vi "Connect Initialize APIs.vi"(0 "Logic VI Ref":refnum<vi>, 5 "SubVIs":refnum<vi>[](array[refnum]), 11 "error in (no error)":errorcluster) -> (15 "error out":errorcluster)   [LabVIEW 2021, in "Migrator.lvlib"]
uses:
  Migrator.lvlib
  Migrator Reusables/Migrator Reusables.lvlib
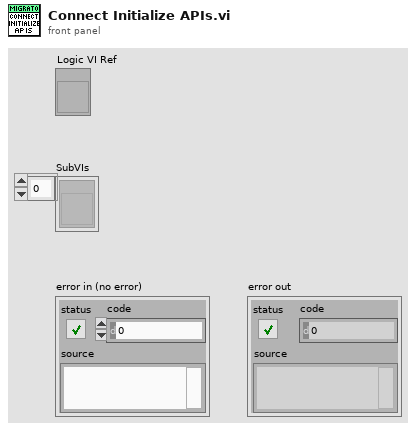
[diagram p1: front panel]
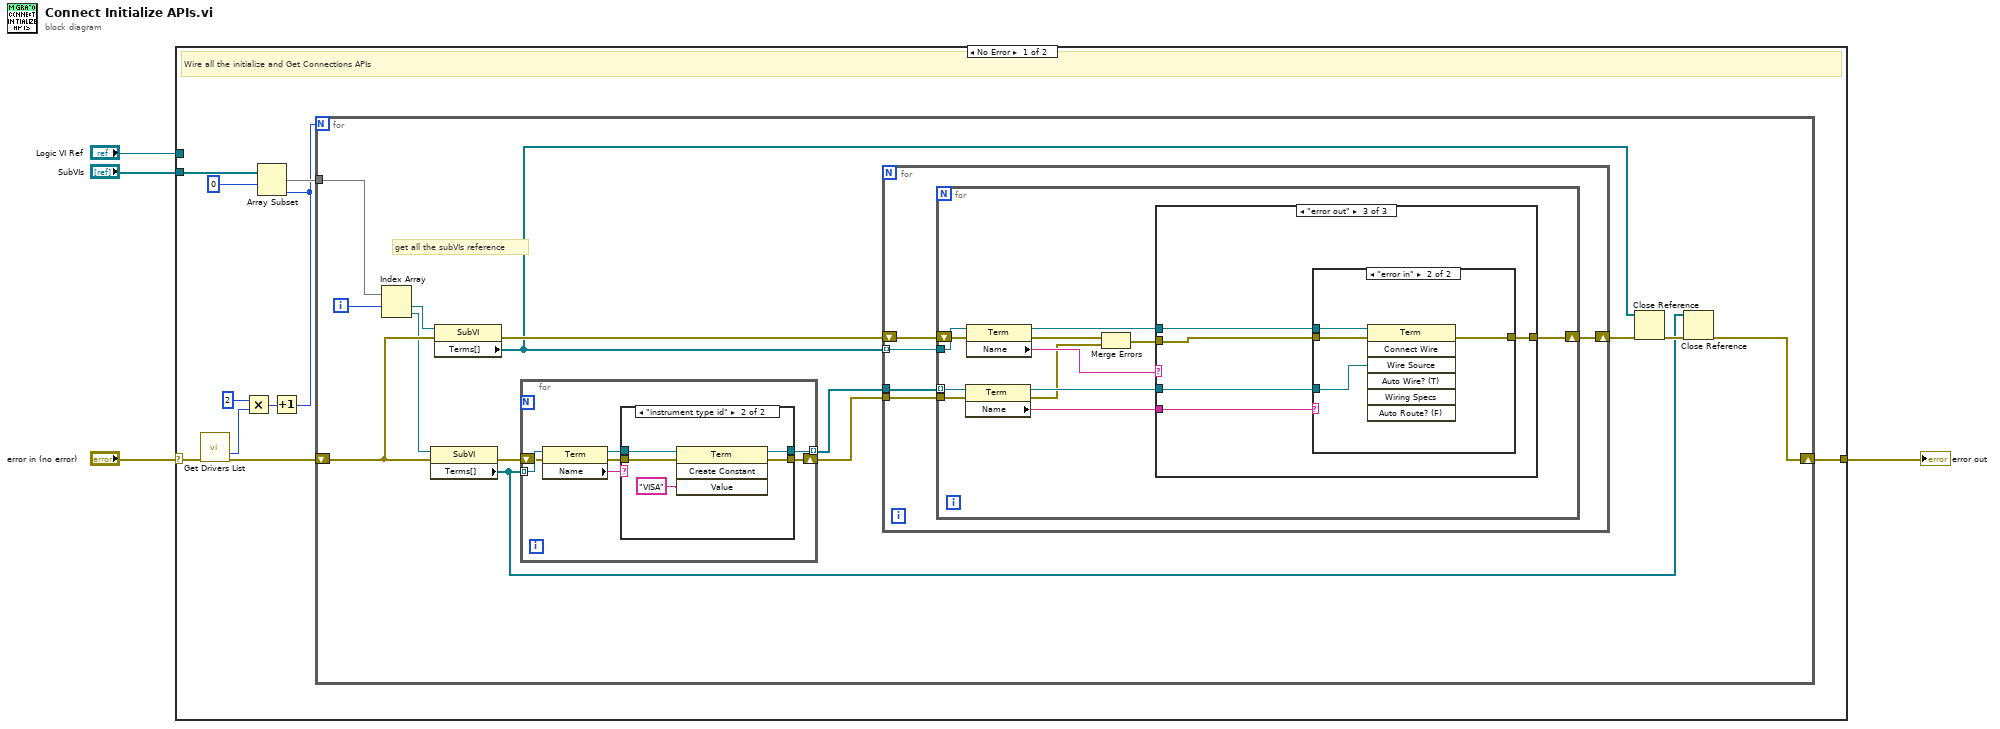
[diagram p0: block diagram]
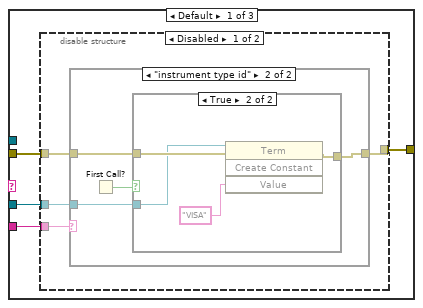
[diagram p3: hidden frame]
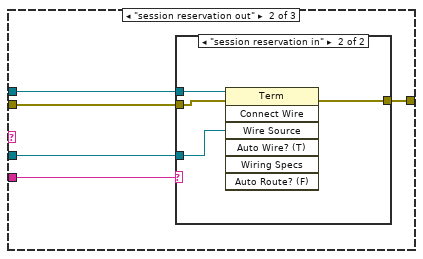
[diagram p7: hidden frame]
diagram:
  n1 = case shown="No Error" "error in (no error)" {
    selector: "error in (no error)" -> [w13 w99]
    tunnel: "Logic VI Ref" -> [_ _]
    tunnel: "SubVIs" -> [w14 _]
    tunnel: [w9 w99] -> w1
    frame No Error {
      # "Wire all the initialize and Get Connections APIs"
      n2 = call "Get Drivers List.vi"("error in (no error)"=w13) -> ("Removed Duplicates Size"=w8:i32, "error out"=w10:errorcluster)  [unwired: 9 in, 4 out]
      n3 = Multiply(x=2, y=w8) -> (x*y=w6:i32)
      n4 = Increment(x=w6) -> (x+1=w5:i32)
      n5 = Array Subset(array=w14, index=0, length=w5) -> (w11:refnum<vi>[])
      n6 = for {
        N: w5 -> [_]
        tunnel: w11 -> [w27]
        shift-right: [w25] -> w9
        shift-left: w10 -> [w26]
        i -> [w28]
        # "get all the subVIs reference"
        n7 = Index Array(array=w27, index #1=w28) -> (element #1=w24:refnum<vi>, element #2=w23:refnum<vi>)  [unwired: 1 in]
        n8 = property class="SubVI"(reference=w23, error in=w26) -> (error out=w18:errorcluster, "Terms[]"=w17:refnum<vi>[])  [unwired: 1 out]
        n9 = property class="SubVI"(reference=w24, error in=w26) -> (error out=w22:errorcluster, "Terms[]"=w20:refnum<vi>[])  [unwired: 1 out]
        n10 = for {
          tunnel: w17 -> [w35] mode=indexing
          tunnel: [w29] -> w15 mode=indexing
          shift-right: [w32] -> w16
          shift-left: w18 -> [w34]
          n11 = property class="Term"(reference=w35, error in=w34) -> (reference out=w30:refnum<vi>, error out=w33:errorcluster, "Name"=w31:string)
          n12 = case shown="\"instrument type id\"" w31 {
            tunnel: w33 -> [w37 w42]
            tunnel: [w37 w41] -> w32
            tunnel: w30 -> [w36 w40]
            tunnel: [w36 w39] -> w29
            frame Default {
            }
            frame "instrument type id" {
              n13 = invoke class="Term" method="Create Constant"(reference=w40, error in=w42, "Value"="VISA") -> (reference out=w39:refnum<vi>, error out=w41:errorcluster)  [unwired: 1 in, 2 out]
            }
          }
        }
        n14 = for {
          tunnel: w20 -> [w46] mode=indexing
          tunnel: w16 -> [w45]
          shift-right: [w44] -> w21
          shift-left: w22 -> [w47]
          tunnel: w15 -> [w43]
          n15 = for {
            tunnel: w46 -> [w58]
            tunnel: w45 -> [w57]
            shift-right: [w49] -> w44
            shift-left: w47 -> [w59]
            tunnel: w43 -> [w48] mode=indexing
            n16 = property class="Term"(reference=w48, error in=w57) -> (reference out=w52:refnum<vi>, error out=w50:errorcluster, "Name"=w55:string)
            n17 = property class="Term"(reference=w58, error in=w59) -> (reference out=w53:refnum<vi>, error out=w54:errorcluster, "Name"=w56:string)
            n18 = Merge Errors(w54, w50) -> (w51:errorcluster)
            n19 = case shown="\"error out\"" w56 {
              tunnel: w55 -> [w63 w83 w93]
              tunnel: w51 -> [w62 w82 w92]
              tunnel: w53 -> [_ w80 w91]
              tunnel: w52 -> [w61 w79 w90]
              tunnel: [w60 w81 w89] -> w49
              frame Default {
                n20 = disable-structure shown="Disabled" {
                  disable-tunnel: w63 -> [w67 _]
                  disable-tunnel: w62 -> [w66 w78]
                  disable-tunnel: w61 -> [w65 _]
                  disable-tunnel: [w64 w78] -> w60
                  frame Disabled {
                    n21 = case shown="\"instrument type id\"" w67 {
                      tunnel: w66 -> [w68 w71]
                      tunnel: w65 -> [_ w70]
                      tunnel: [w68 w69] -> w64
                      frame Default {
                      }
                      frame "instrument type id" {
                        n22 = First Call?() -> (First Call?: T/F=w72:bool)
                        n23 = case shown="True" w72 {
                          tunnel: w71 -> [w73 w77]
                          tunnel: w70 -> [_ w76]
                          tunnel: [w73 w74] -> w69
                          frame False {
                          }
                          frame True {
                            n24 = invoke class="Term" method="Create Constant"(reference=w76, error in=w77, "Value"="VISA") -> (error out=w74:errorcluster)  [unwired: 1 in, 3 out]
                          }
                        }
                      }
                    }
                  }
                  frame Enabled {
                  }
                }
              }
              frame "session reservation out" {
                n25 = case shown="\"session reservation in\"" w83 {
                  tunnel: w82 -> [w84 w87]
                  tunnel: [w84 w85] -> w81
                  tunnel: w80 -> [_ w88]
                  tunnel: w79 -> [_ w86]
                  frame Default {
                  }
                  frame "session reservation in" {
                    n26 = invoke class="Term" method="Connect Wire"(reference=w88, error in=w87, "Wire Source"=w86) -> (error out=w85:errorcluster)  [unwired: 4 in, 6 out]
                  }
                }
              }
              frame "error out" {
                n27 = case shown="\"error in\"" w93 {
                  tunnel: w92 -> [w94 w96]
                  tunnel: w91 -> [_ w98]
                  tunnel: w90 -> [_ w97]
                  tunnel: [w94 w95] -> w89
                  frame Default {
                  }
                  frame "error in" {
                    n28 = invoke class="Term" method="Connect Wire"(reference=w98, error in=w96, "Wire Source"=w97) -> (error out=w95:errorcluster)  [unwired: 4 in, 6 out]
                  }
                }
              }
            }
          }
        }
        n29 = Close Reference(reference=w20, error in (no error)=w21) -> (error out=w19:errorcluster)
        n30 = Close Reference(reference=w17, error in (no error)=w19) -> (error out=w25:errorcluster)
      }
    }
    frame Error {
    }
  }
  "error out" <- w1
